vi "NewDiagPacketArrivedCallback.vi"(4 "ControllerDiagPacket":refnum<user-event>, 5 "Event Data":T1, 6 "Control Ref":refnum<k24>, 7 "Event Common Data":T2) -> ()   [LabVIEW 2019]
uses:
  C:/Users/patrick/Documents/GitHub/Aerotech-Delay-Line/lvsrc/Aerotech-Ensemble-LabVIEW/2010-5.6/Bin/Aerotech.Ensemble.LabVIEW.dll
  Bin/Aerotech.Ensemble.LabVIEW.dll
  C:/Users/patrick/Documents/GitHub/Aerotech-Delay-Line/lvsrc/Aerotech-Ensemble-LabVIEW/2010-5.6/Bin/Aerotech.Ensemble.dll
  Bin/Aerotech.Ensemble.dll
  ControllerDiagPacket.ctl
  AxisDiagPacket.ctl
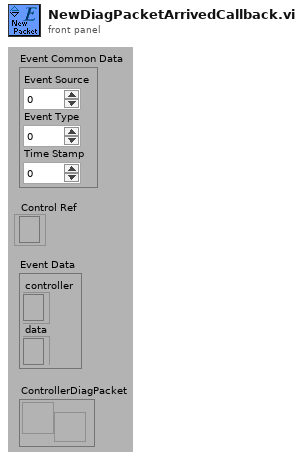
[diagram p1: front panel]
types:
  T1 = cluster{"controller":refnum<k24>, "data":refnum<k24>}
  T2 = cluster{"Event Source":i32, "Event Type":u32, "Time Stamp":u32}
  T3 = typedef "ControllerDiagPacket.ctl" = cluster{"Count":i32, "Packet Time":i64, "Axes":T4[], "error":errorcluster}
  T4 = typedef "AxisDiagPacket.ctl" = cluster{"Axis Name":string, "Acceleration Command":dbl, "Amplifier Temperature":sgl, "Analog Input 0":dbl, "Analog Input 1":dbl, "Analog Output 0":dbl, "Analog Output 1":dbl, "Axis Fault (num)":i32, "Axis Fault (str)":string, "Axis Fault (bits)":cluster{"AmplifierFault":bool, "AmplifierTemperatureFault":bool, "CcwEndOfTravelLimitFault":bool, "CcwSoftwareLimitFault":bool, "CommunicationLostFault":bool, "CwEndOfTravelLimitFault":bool, "CwSoftwareLimitFault":bool, "EmergencyStopFault":bool, "EncoderFault":bool, "ExternalFault":bool, "FeedbackScalingFault":bool, "HallSensorFault":bool, "MarkerSearchFault":bool, "MaxVelocityCommandFault":bool, "MotorTemperatureFault":bool, "None":bool, "OverCurrentFault":bool, "PositionErrorFault":bool, "PositionFeedbackFault":bool, "PowerSupplyFault":bool, "VelocityErrorFault":bool, "VelocityFeedbackFault":bool, "VoltageClampFault":bool}, "Axis Status (num)":i32, "Axis Status (str)":string, "Axis Status (bits)":cluster{"AccelerationPhase":bool, "AutofocusActive":bool, "BrakeOutput":bool, "CalibrationActive":bool, "CalibrationEnabled":bool, "CcwEndOfTravelLimitInput":bool, "CommandShapingFilterDone":bool, "CosineEncoderError":bool, "CurrentClamp":bool, "CwEndOfTravelLimitInput":bool, "DecelerationPhase":bool, "EmergencyStopInput":bool, "Enabled":bool, "GantryMasterActive":bool, "GantryModeActive":bool, "HallAInput":bool, "HallBInput":bool, "HallCInput":bool, "Homed":bool, "HomeLimitInput":bool, "Homing":bool, "InPosition":bool, "InPosition2":bool, "JoystickControl":bool, "MarkerInput":bool, "MasterMotionSuppressed":bool, "MasterSlaveControl":bool, "MotionIsCw":bool, "MoveActive":bool, "None":bool, "PositionCaptureActive":bool, "ServoControl":bool, "SineEncoderError":bool}, "Current Command":sgl, "Current Error":sgl, "Current Feedback":sgl, "Digital Input 0":i32, "Digital Input 1":i32, "Digital Input 2":i32, "Digital Output 0":i32, "Digital Output 1":i32, "Digital Output 2":i32, "Position Feedback Auxiliary":dbl, "Position Command":dbl, "Position Error":dbl, "Position Feedback":dbl, "Program Position Command":dbl, "Program Position Error":dbl, "Program Position Feedback":dbl, "Velocity Command":dbl, "Velocity Error":dbl, "Velocity Feedback":dbl}
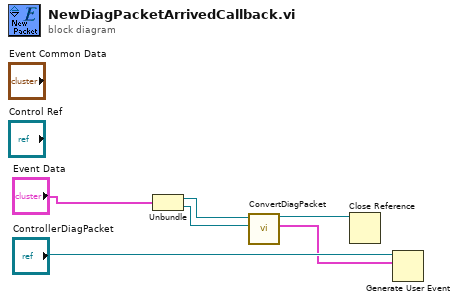
[diagram p0: block diagram]
diagram:
  n1 = Unbundle("Event Data") -> ("controller"=w2:refnum<k24>, "data"=w3:refnum<k24>)
  n2 = call "ConvertDiagPacket.vi"(".NET data in"=w3, "controller in"=w2) -> ("LabVIEW data out"=w4:T3, "controller out"=w1:refnum<k24>)  [unwired: 7 in, 1 out]
  n3 = Close Reference(reference=w1) -> ()  [unwired: 1 in, 1 out]
  n4 = Generate User Event(user event="ControllerDiagPacket", event data cluster=w4) -> ()  [unwired: 2 in, 2 out]
